vi "ex6-9.vi"   [LabVIEW 2013]
uses:
  <vilib>/NXT/Block Support/NXT_InputPort.ctl
types:
  T1 = typedef "LVHSConnector.ctl" = refnum<class "BrickReference.lvclass">
  T2 = typedef "NXT_InputPort.ctl" = u32
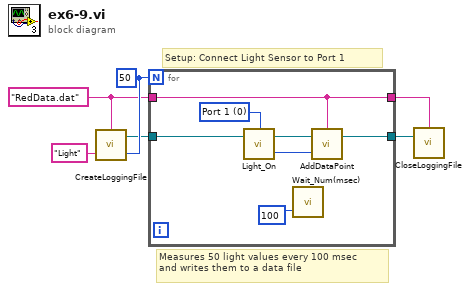
[diagram p0: block diagram]
diagram:
  w6 = u32 50 ("milliseconds to wait")
  w2 = "RedData.dat" ("Filename")
  # "Measures 50 light values every 100 msec \nand writes them to a data file"
  # "Setup: Connect Light Sensor to Port 1"
  n1 = call <vilib>:"CreateLoggingFile.vi"("Sensor Name"="Light" ("Sensor(s) Name"), "Number of Points"=w6, "Filename"=w2) -> ("NXT/EV3"=w1:T1)  [unwired: 1 in]
  n2 = for {
    N: w6 -> [_]
    tunnel: w2 -> [w10]
    tunnel: [w10] -> w5
    tunnel: w1 -> [w9]
    tunnel: [w13] -> w4
    w7 = T2 0 items=["Port 1", "Port 2", "Port 3", "Port 4"] ("Port (Port 4)")
    n3 = call <vilib>:"Light_On.vi"("NXT/EV3"=w9, "Port (Port 3)"=w7) -> ("Scaled Value"=w11:i16, "NXT/EV3"=w12:T1)  [unwired: 1 in]
    n4 = call <vilib>:"Wait_Num(msec).vi"("Time (100 msec)"=u32 100 ("milliseconds to wait")) -> ()  [unwired: 3 in, 1 out]
    n5 = call <vilib>:"AddDataPoint.vi"("Value"=w11, "NXT/EV3"=w12, "Filename"=w10) -> ("NXT/EV3"=w13:T1)  [unwired: 1 in]
  }
  n6 = call <vilib>:"CloseLoggingFile.vi"("NXT/EV3"=w4, "Filename"=w5) -> ()  [unwired: 2 in, 1 out]
